vi "WD_Block_Move.vi"(7 "站點(記錄用)":string="790", 8 "error in (no error)":errorcluster, 10 "Workplace_id":i16, 11 "DBLink":string) -> (2 "workplace_data":cluster{"條碼R":string, "條碼L":string})   [LabVIEW 2019]
panel:
  # "此id為該位置檔快放行，把資料移至移動中"
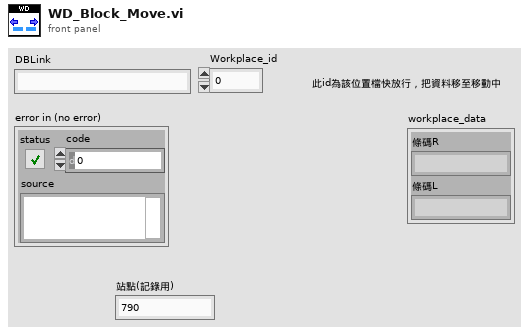
[diagram p1: front panel]
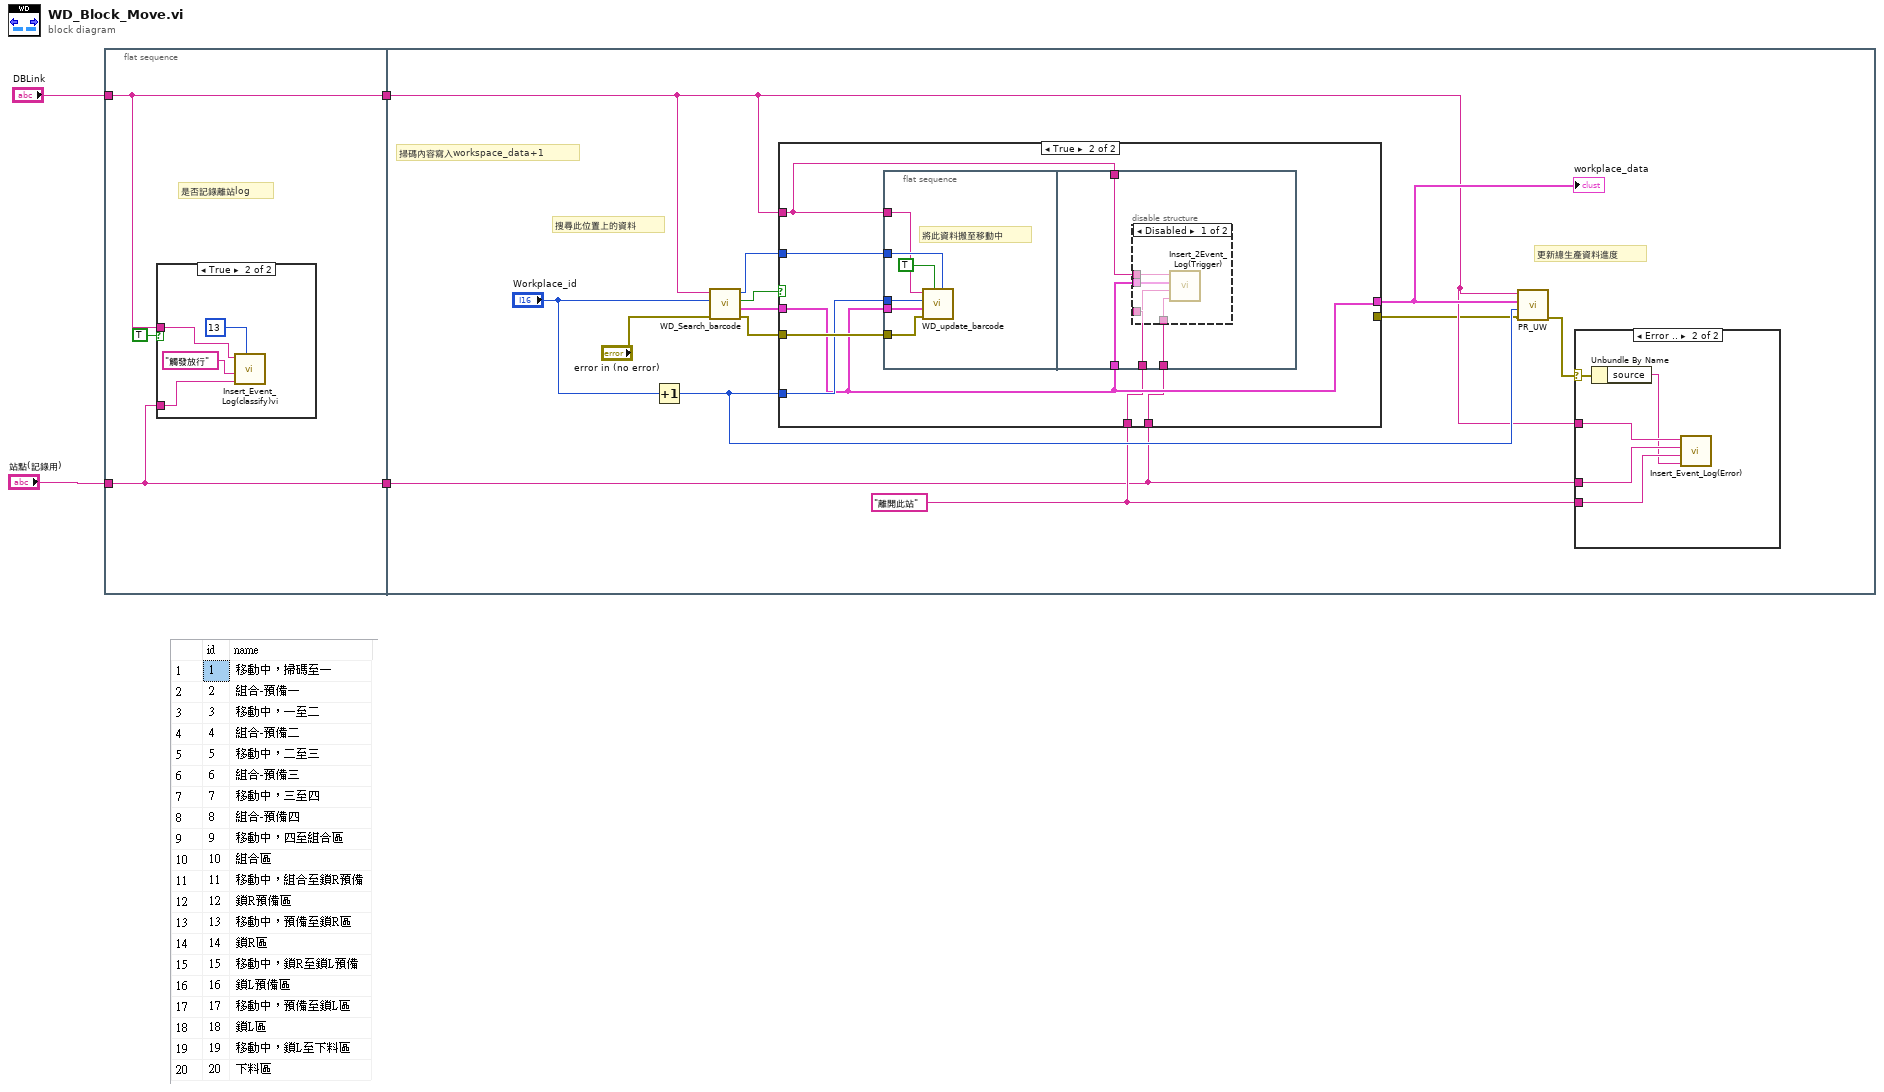
[diagram p0: block diagram]
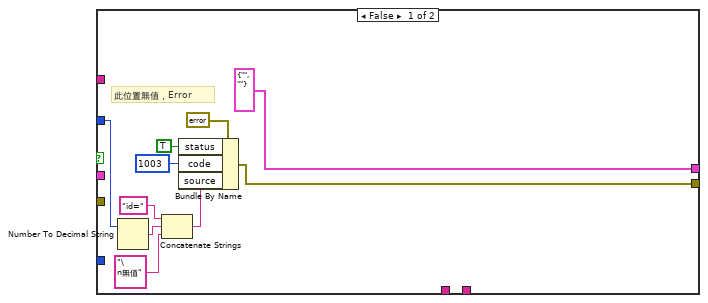
[diagram p4: hidden frame]
diagram:
  n1 = flat-sequence {
    tunnel: "站點(記錄用)" -> [w6]
    tunnel: "DBLink" -> [w7]
    tunnel: [w7] -> w2
    tunnel: [w6] -> w1
    tunnel: w2 -> [w15]
    tunnel: w1 -> [w13]
    frame #0 {
      # "是否記錄離站log"
      n2 = case shown="True" TRUE {
        tunnel: w7 -> [_ w9]
        tunnel: w6 -> [_ w8]
        frame False {
        }
        frame True {
          n3 = call "Insert_Event_Log(classify)vi.vi"("classify"=i16 13, "data"=w8, "message"="觸發放行", "DBlink"=w9) -> ()  [unwired: 7 in, 1 out]
        }
      }
    }
    frame #1 {
      w14 = "離開此站" ("message")
      # "搜尋此位置上的資料"
      # "更新總生產資料進度"
      # "掃碼內容寫入workspace_data+1"
      n4 = Increment(x="Workplace_id") -> (x+1=w18:i16)
      n5 = call "WD_Search_barcode.vi"("error in (no error)"="error in (no error)", "workplace_name_id"="Workplace_id", "DBlink"=w15) -> ("error out"=w23:errorcluster, "workplace_data"=w22:cluster{"條碼R":string, "條碼L":string}, "找到"=w21:bool, "取得ID"=w24:i16)  [unwired: 5 in]
      n6 = case shown="True" w21 {
        tunnel: w15 -> [_ w42]
        tunnel: w22 -> [_ w43]
        tunnel: w23 -> [_ w46]
        tunnel: w24 -> [w36 w45]
        tunnel: w18 -> [_ w44]
        tunnel: [cluster{"條碼A":string, "條碼B":string} {"條碼A"="", "條碼B"=""} ("workplace_data") w43] -> w17
        tunnel: w13 -> [_ w41]
        tunnel: w14 -> [_ w40]
        tunnel: [w30 _] -> w12
        frame False {
          # "此位置無值，Error"
          n7 = Number To Decimal String(number=w36) -> (decimal integer string=w34:string)  [unwired: 1 in]
          n8 = Concatenate Strings("id=", w34, "\n無值" ("string")) -> (w32:string)
          n9 = Bundle By Name(cluster=errorcluster {"status"=FALSE, "code"=0, "source"=""} ("error out"), "status"=TRUE, "code"=1003, "source"=w32) -> (w30:errorcluster)
        }
        frame True {
          n10 = flat-sequence {
            tunnel: w46 -> [w52]
            tunnel: w45 -> [w50]
            tunnel: w44 -> [w49]
            tunnel: w42 -> [w48]
            tunnel: w43 -> [w47]
            tunnel: w43 -> [w56]
            tunnel: w42 -> [w55]
            tunnel: w41 -> [w54]
            tunnel: w40 -> [w53]
            frame #0 {
              # "將此資料搬至移動中"
              n11 = call "WD_update_barcode.vi"("NULL: workplace_id"=w50, "Set null"=TRUE, "error in (no error)"=w52, "Workplace data"=w47, "workplace_id"=w49, "DBlink"=w48) -> ()  [unwired: 6 in]
            }
            frame #1 {
              n12 = disable-structure shown="Disabled" {
                disable-tunnel: w56 -> [w60 _]
                disable-tunnel: w55 -> [w59 _]
                disable-tunnel: w54 -> [w58 _]
                disable-tunnel: w53 -> [w57 _]
                frame Disabled {
                  n13 = call "Insert_2Event_Log(Trigger).vi"("data"=w58, "message"=w57, "output cluster"=w60, "DBlink"=w59) -> ()  [unwired: 8 in]
                }
                frame Enabled {
                }
              }
            }
          }
        }
      }
      "workplace_data" <- w17
      n14 = call "PR_UW .vi"("error in (no error)"=w12, "[workplace_id]"=w18, "當前工位資料"=w17, "DBlink"=w15) -> ("error out"=w16:errorcluster)  [unwired: 7 in]
      n15 = case shown="Error .." w16 {
        selector: w16 -> [_ w26]
        tunnel: w15 -> [_ w29]
        tunnel: w13 -> [_ w28]
        tunnel: w14 -> [_ w27]
        frame No Error {
        }
        frame Error {
          n16 = Unbundle By Name(w26) -> ("source"=w25:string)
          n17 = call "Insert_Event_Log(Error).vi"("data"=w25, "message"=w27, "id"=w28, "DBlink"=w29) -> ()  [unwired: 8 in]
        }
      }
    }
  }
